vi "InitializeScanEngine.vi"(8 "error in (no error)":errorcluster, 11 "Qbus":refnum<class "Qbus.lvclass">) -> (0 "error out":errorcluster, 2 "valid":bool, 3 "scan engine config":T1)   [LabVIEW 2017, in "ScanEngine.lvlib"]
uses:
  <vilib>/addons/InsightCM/Devices/Shared/Common/ScanEngine/ScanEngine.lvlib
  <vilib>/addons/InsightCM/Devices/Shared/Common/ScanEngine/controls/Configuration.ctl
  <vilib>/addons/InsightCM/Devices/Shared/Common/ScanEngine/controls/Group.ctl
  <vilib>/addons/InsightCM/Devices/Shared/Common/ScanEngine/controls/Channel.ctl
  <vilib>/Utility/Data Type/Type Definitions/Data Type.ctl
  <vilib>/addons/InsightCM/MessageBus/Base/controls/KeyValuePair.ctl
  <vilib>/addons/Qbus/Qbus.lvclass
  <vilib>/addons/InsightCM/Utilities/GlobalConfiguration/GlobalConfiguration.lvlib
  <vilib>/addons/InsightCM/Devices/Shared/Common/DataEventCreator/DataEventCreator.lvlib
  <vilib>/addons/InsightCM/Devices/Shared/Cms/CmsDataEventCreator/CmsDataEventCreator.lvlib
  <vilib>/Utility/Data Type/NI_Data Type.lvlib
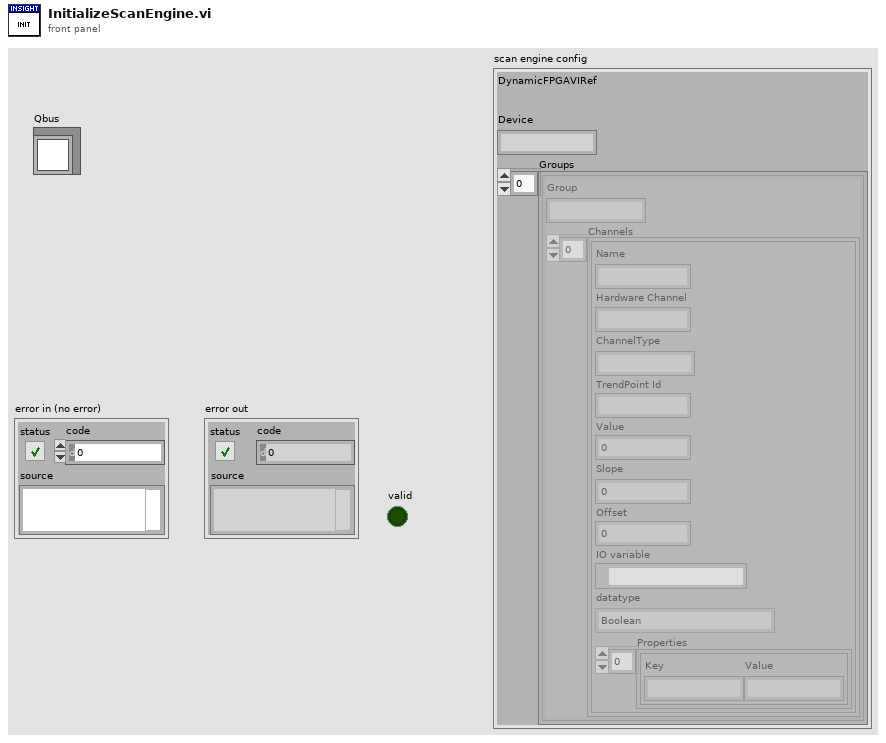
[diagram p1: front panel]
types:
  T1 = typedef "ScanEngine.lvlib/Configuration.ctl" = cluster{"DynamicFPGAVIRef":refnum<k20>, "Device":string, "Groups":T2[]}
  T2 = typedef "ScanEngine.lvlib/Group.ctl" = cluster{"Group":string, "Channels":T3[]}
  T3 = typedef "ScanEngine.lvlib/Channel.ctl" = cluster{"Name":string, "Hardware Channel":string, "ChannelType":string, "TrendPoint Id":string, "Value":sgl, "Slope":dbl, "Offset":dbl, "IO variable":refnum<k21>, "datatype":T4, "Properties":T5[]}
  T4 = typedef "NI_Data Type.lvlib/Data Type.ctl" = enum8{"Invalid Type", "Void", "I8", "I16", "I32", "I64", "U8", "U16", "U32", "U64", "Single Float", "Double Float", "Extended Float", "Single Complex", "Double Complex", "Extended Complex", "Enum U8", "Enum U16", "Enum U32", "Enum U64", "Single Float With Unit", "Double Float With Unit", "Extended Float With Unit", "Single Complex with Unit", "Double Complex with Unit", "Extended Complex with Unit", "Boolean", "String", "Path", "Picture", "Tag", "Array", "Cluster", "Variant", "LV Variant", "Waveform", "Timestamp", "Digital Waveform", "Digital Data", "ExpressData", "Refnum", "External Data", "VI", "Poly VI", "LabVIEW Class Instance", "Fixed Point"}
  T5 = typedef "KeyValuePair.ctl" = cluster{"Key":string, "Value":string}
  T6 = typedef "AssetNode.ctl" = cluster{"Id":string, "Type":string, "Name":string, "ParentIds":string[], "State":T7, "MeasType":string, "Properties":T5[], "OperatingStates":T8[], "Metrics":T11[], "TrendAlarmRules":T12[], "References":T15[]}
  T7 = typedef "AssetState.ctl" = cluster{"Disabled":bool}
  T8 = typedef "OperatingState.ctl" = cluster{"Name":string, "Properties":T5[], "Triggers":T9[]}
  T9 = typedef "Trigger.ctl" = cluster{"Type":string, "Expression":string, "Conditions":T10[]}
  T10 = typedef "Condition.ctl" = cluster{"Source":string, "Type":string, "Operator":string, "CompareTo":string, "DwellSeconds":dbl}
  T11 = typedef "Metric.ctl" = cluster{"Id":string, "Name":string, "Unit":string, "Properties":T5[], "MetricDefinitionInstanceId":string}
  T12 = typedef "TrendAlarmRule.ctl" = cluster{"Id":string, "AssetNodeId":string, "TrendId":string, "Disabled":bool, "OperatingState":string, "Operator":string, "Hysteresis":dbl, "OnDelaySeconds":dbl, "OffDelaySeconds":dbl, "Levels":T13[], "Properties":T5[]}
  T13 = typedef "TrendAlarmLevel.ctl" = cluster{"Severity":i32, "CompareTo":dbl, "Actions":T14[]}
  T14 = typedef "AlarmAction.ctl" = cluster{"Type":string, "Props":T5[]}
  T15 = typedef "AssetNodeReference.ctl" = cluster{"NodeId":string, "Name":string}
  T16 = typedef "R2_Device.ctl" = cluster{"Id":string, "Name":string, "DeviceType":string, "HardwareName":string, "IpAddress":string, "HardwareInfo":T5[], "ApplicationType":string, "ApplicationVersion":string, "EquipmentIds":string[], "ConfigurationVersion":string, "State":T17, "Properties":T5[], "DataGroups":T18[], "BurstModeTrigger":T19}
  T17 = typedef "DeviceState.ctl" = cluster{"Disabled":bool}
  T18 = typedef "R2_DataGroup.ctl" = cluster{"Name":string, "OperatingStates":T8[], "Properties":T5[], "EquipmentIds":string[], "AssetNodeId":string}
  T19 = typedef "BurstModeTrigger.ctl" = cluster{"Trigger":T9, "SampleRate":string, "AcquisitionLength":string}
  T20 = typedef "R2_Channel.ctl" = cluster{"Id":string, "DeviceId":string, "Name":string, "ChannelType":string, "HardwareKey":string, "HardwareChannel":string, "DataGroup":string, "Keywords":string[], "EquipmentIds":string[], "Properties":T5[], "Metrics":T11[], "AssetNodeId":string, "MeasType":string, "AssetName":string}
  T21 = typedef "DataEventCreator.lvlib/RegisterTrendPoints.ctl" = cluster{"DataGroup":string, "Trends":T22[]}
  T22 = typedef "DataEventCreator.lvlib/Registry_Trend.ctl" = cluster{"TrendPointId":string, "DataSetName":string, "HighRate":bool, "Always Send":bool}
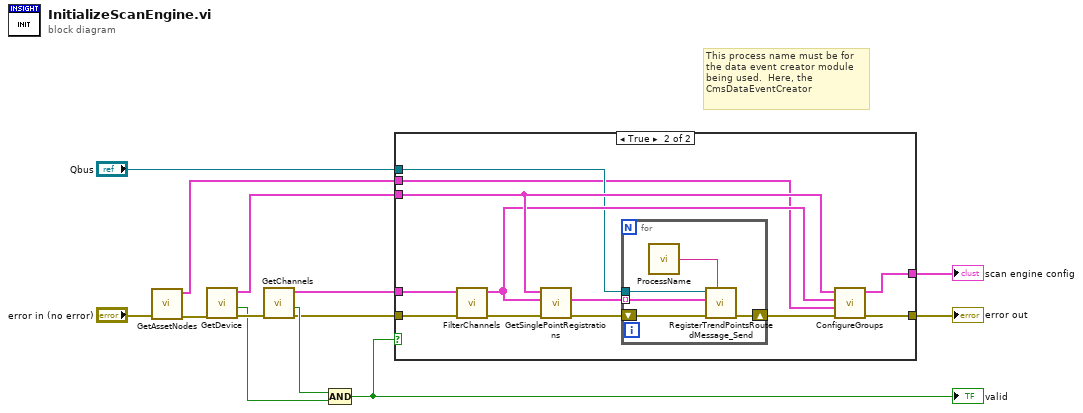
[diagram p0: block diagram]
diagram:
  # "This process name must be for\nthe data event creator module\nbeing used.  Here, the \nCmsDataEventCreator"
  n1 = call <vilib>:"GetAssetNodes.vi"("error in (no error)"="error in (no error)") -> ("error out"=w2:errorcluster, "AssetNodes"=w1:T6[])  [unwired: 8 in, 1 out]
  n2 = call <vilib>:"GetDevice.vi"("error in (no error)"=w2) -> ("error out"=w11:errorcluster, "found"=w10:bool, "device configuration"=w12:T16)  [unwired: 8 in]
  n3 = call <vilib>:"GetChannels.vi"("error in (no error)"=w11) -> ("error out"=w4:errorcluster, "found"=w9:bool, "channels"=w13:T20[])  [unwired: 8 in]
  n4 = Compound Arithmetic op=AND(w9, w10) -> (w5:bool)
  "valid" <- w5
  n5 = case shown="True" w5 {
    tunnel: w13 -> [_ w20]
    tunnel: w12 -> [_ w26]
    tunnel: w4 -> [w14 w25]
    tunnel: [w14 w16] -> w8
    tunnel: [_ w23] -> w7
    tunnel: "Qbus" -> [_ w17]
    tunnel: w1 -> [_ w15]
    frame False {
    }
    frame True {
      n6 = call <vilib>:"FilterChannels.vi"("error in (no error)"=w25, "channels"=w20) -> ("error out"=w24:errorcluster, "single point channels"=w19:T20[])  [unwired: 8 in]
      n7 = call <vilib>:"GetSinglePointRegistrations.vi"("error in (no error)"=w24, "single point channels"=w19, "device"=w26) -> ("error out"=w21:errorcluster, "register trends"=w22:T21[])  [unwired: 7 in]
      n8 = for {
        tunnel: w22 -> [w29] mode=indexing
        shift-right: [w30] -> w18
        shift-left: w21 -> [w31]
        tunnel: w17 -> [w28]
        n9 = call <vilib>:"ProcessName.vi"() -> ("process name"=w27:string)  [unwired: 5 in]
        n10 = call <vilib>:"RegisterTrendPointsRoutedMessage_Send.vi"("data event creator process name"=w27, "error in (no error)"=w31, "register trend"=w29, "Qbus in"=w28) -> ("error out"=w30:errorcluster)  [unwired: 6 in, 1 out]
      }
      n11 = call <vilib>:"ConfigureGroups.vi"("error in (no error)"=w18, "AssetNodes"=w15, "single point channels"=w19, "device"=w26) -> ("error out"=w16:errorcluster, "config"=w23:T1)  [unwired: 6 in]
    }
  }
  "scan engine config" <- w7
  "error out" <- w8
